vi "Msg To.vi"() -> (3 "Teardown Msg Strategy out":refnum<class "Teardown Msg Strategy.lvclass">)   [LabVIEW 2021, in "jettl.lvlib" / "Teardown.lvlib" / "Teardown Msg Strategy.lvclass"]
uses:
  Teardown Msg Strategy.lvclass
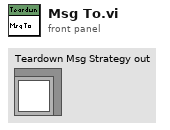
[diagram p1: front panel]
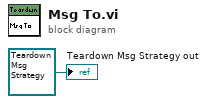
[diagram p0: block diagram]
diagram:
  "Teardown Msg Strategy out" <- refnum<class "Teardown Msg Strategy.lvclass"> refnum ("Destroy Msg in")
